vi "Get ListObj.vi"(8 "error in (no error)":errorcluster, 11 "StringList in":refnum<class "StringList.lvclass">) -> (0 "error out":errorcluster, 2 "List Object":refnum<class "List.lvclass">, 3 "StringList out":refnum<class "StringList.lvclass">)   [LabVIEW 2017, in "LapDog.Collections.v0.Lists.Interfaces.lvlib" / "StringList.lvclass"]
uses:
  StringList.lvclass
  Lists/List/List.lvclass
  StringList.lvclass/StringList.ctl
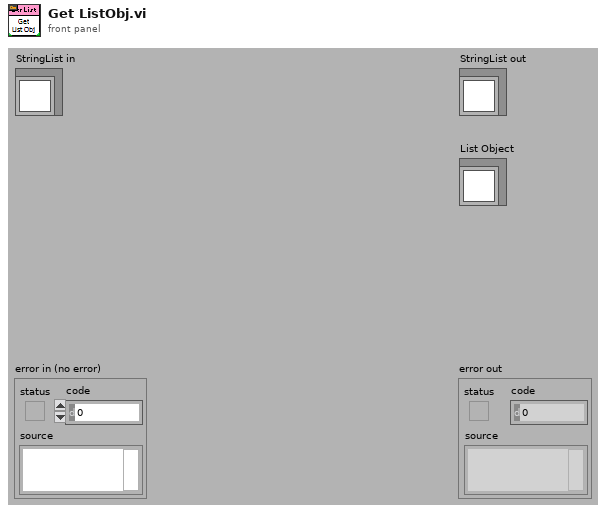
[diagram p1: front panel]
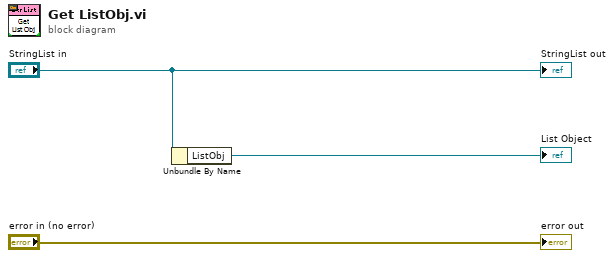
[diagram p0: block diagram]
diagram:
  n1 = Unbundle By Name("StringList in") -> ("ListObj"=→"List Object":refnum<class "List.lvclass">)
  "error out" <- "error in (no error)"
  "StringList out" <- "StringList in"
